vi "Read Digital Out Status.vi"(8 "error in":errorcluster, 11 "MiniIO in":refnum<class "MiniIO.lvclass">) -> (0 "error out":errorcluster, 3 "MiniIO out":refnum<class "MiniIO.lvclass">)   [LabVIEW 2018, in "MiniIO.lvlib" / "MiniIO.lvclass"]
uses:
  MiniIO.lvclass
  MiniIO.lvclass/MiniIO.ctl
  <vilib>/NI/Modbus Library/API/Master/Modbus Master.lvclass
  PPLs/PLC/Parent/PLC.lvlibp/PLC.lvclass
  C:/AME Test Engineering/LabVIEW/PPLs/PLC/Parent/PLC.lvlibp/PLC.lvclass
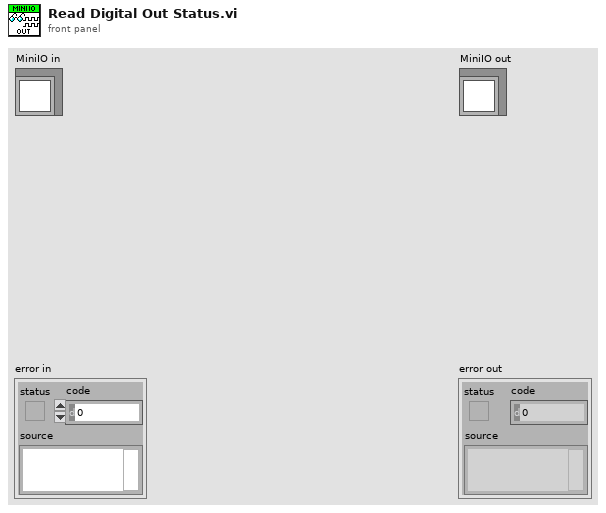
[diagram p1: front panel]
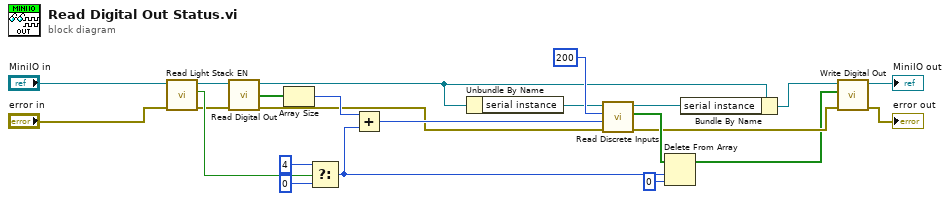
[diagram p0: block diagram]
diagram:
  n1 = call "Read Light Stack EN.vi"("error in (no error)"="error in", "PLC in"="MiniIO in") -> ("error out"=w7:errorcluster, "Light Stack?"=w9:bool, "PLC out"=w8:refnum<class "MiniIO.lvclass">)  [unwired: 7 in]
  n2 = call "Read Digital Out.vi"("error in"=w7, "PLC in"=w8) -> ("error out"=w5:errorcluster, "Digital Out"=w6:bool[], "PLC out"=w2:refnum<class "MiniIO.lvclass">)  [unwired: 7 in]
  n3 = Array Size(array=w6) -> (size(s)=w23:i32)
  n4 = Select(t=4 ("index"), s=w9, f=0 ("index")) -> (s? t:f=w16:i32)
  n5 = Add(x=w23, y=w16) -> (x+y=w17:i32)
  n6 = Unbundle By Name(w2) -> ("serial instance"=w1:refnum<class "Modbus Master.lvclass">)
  n7 = call-dynamic "Read Discrete Inputs.vi"("error in"=w5, "number of inputs"=w17, "starting address"=u16 200, "Modbus master in"=w1) -> ("error out"=w4:errorcluster, "discrete inputs"=w21:bool[], "Modbus master out"=w12:refnum<class "Modbus Master.lvclass">)  [unwired: 5 in]
  n8 = Delete From Array(array=w21, length=w16, index=0) -> (array with subset deleted=w3:bool[])  [unwired: 1 out]
  n9 = Bundle By Name(cluster=w2, "serial instance"=w12) -> (w15:refnum<class "MiniIO.lvclass">)
  n10 = call "Write Digital Out.vi"("error in (no error)"=w4, "Digital Out"=w3, "PLC in"=w15) -> ("error out"=→"error out":errorcluster, "PLC out"=→"MiniIO out":refnum<class "MiniIO.lvclass">)  [unwired: 7 in]
